vi "digitalOutput.vi"(0 "valve data":bool[](array[boolean])=[FALSE, FALSE, FALSE, FALSE, FALSE, FALSE, FALSE, FALSE]) -> ()   [LabVIEW 2011]
uses:
  GlobalDAQ.vi
  <vilib>/ULx/Write.llb/ULx Write (Digital 1D Bool 1Chan 1Samp).vi
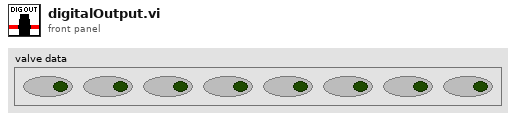
[diagram p1: front panel]
types:
  T1 = typedef "Semaphore RefNum" = refnum<k1>
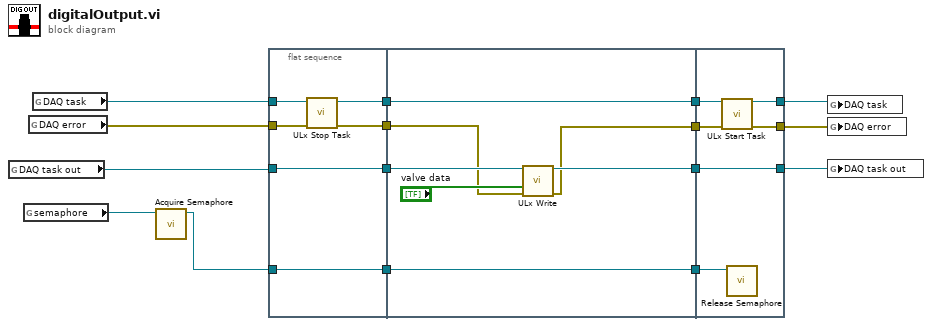
[diagram p0: block diagram]
diagram:
  n1 = global read "GlobalDAQ.vi" "DAQ task out"() -> (w5:refnum<k24>)
  n2 = global read "GlobalDAQ.vi" "semaphore"() -> (w4:T1)
  n3 = global read "GlobalDAQ.vi" "DAQ error"() -> (w12:errorcluster)
  n4 = global read "GlobalDAQ.vi" "DAQ task"() -> (w16:refnum<k24>)
  n5 = call <vilib>:"Acquire Semaphore.vi"("semaphore"=w4) -> ("semaphore out"=w2:T1)  [unwired: 4 in, 2 out]
  n6 = flat-sequence {
    tunnel: w16 -> [w22]
    tunnel: [w21] -> w14
    tunnel: w12 -> [w20]
    tunnel: [w19] -> w11
    tunnel: w5 -> [w19]
    tunnel: [w18] -> w8
    tunnel: [w17] -> w3
    tunnel: w2 -> [w17]
    tunnel: [w29] -> w15
    tunnel: w14 -> [w29]
    tunnel: w11 -> [w28]
    tunnel: [w27] -> w10
    tunnel: w8 -> [w25]
    tunnel: [w24] -> w7
    tunnel: w3 -> [w23]
    tunnel: [w23] -> w1
    tunnel: w15 -> [w35]
    tunnel: [w34] -> w13
    tunnel: [w33] -> w9
    tunnel: w10 -> [w33]
    tunnel: w7 -> [w32]
    tunnel: [w31] -> w6
    tunnel: w1 -> [w30]
    frame #0 {
      n7 = call <vilib>:"ULx Stop Task.vi"("error in"=w20, "task in"=w22) -> ("error out"=w18:errorcluster, "task out"=w21:refnum<k24>)  [unwired: 8 in]
    }
    frame #1 {
      n8 = call-poly <vilib>:"ULx Write.vi"("task in"=w28, "data"="valve data", "error in"=w25) -> ("task out"=w27:refnum<k24>, "error out"=w24:errorcluster)  [unwired: 10 in, 1 out]
    }
    frame #2 {
      n9 = call <vilib>:"ULx Start Task.vi"("task in"=w35, "error in"=w32) -> ("task out"=w34:refnum<k24>, "error out"=w31:errorcluster)  [unwired: 12 in]
      n10 = call <vilib>:"Release Semaphore.vi"("semaphore"=w30) -> ()  [unwired: 5 in, 2 out]
    }
  }
  n11 = global write "GlobalDAQ.vi" "DAQ task"(w13) -> ()
  n12 = global write "GlobalDAQ.vi" "DAQ error"(w6) -> ()
  n13 = global write "GlobalDAQ.vi" "DAQ task out"(w9) -> ()
